vi "TestExec.Lookup Sequence XML Result Folder.vi"(9 "Seq Result Dirs":T1[](array[typedef]), 10 "Default Result Folder":path, 11 "Seq Name":string) -> (2 "None":bool, 3 "Result Folder":path)   [LabVIEW 2018]
uses:
  Common/Utils/TestExec/TestExec.WorkingDir.ctl
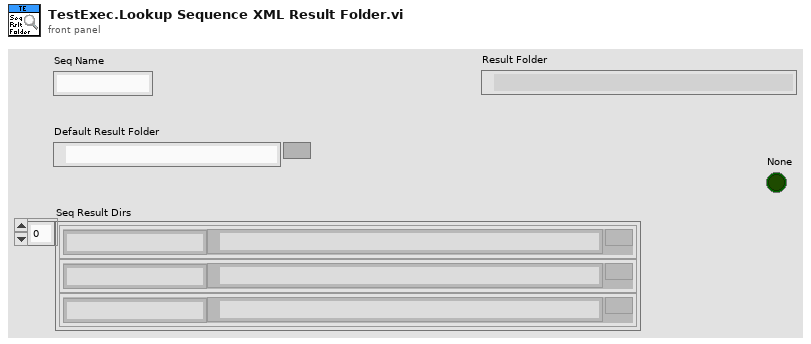
[diagram p1: front panel]
types:
  T1 = typedef "TestExec.WorkingDir.ctl" = cluster{"Name":string, "Path":path}
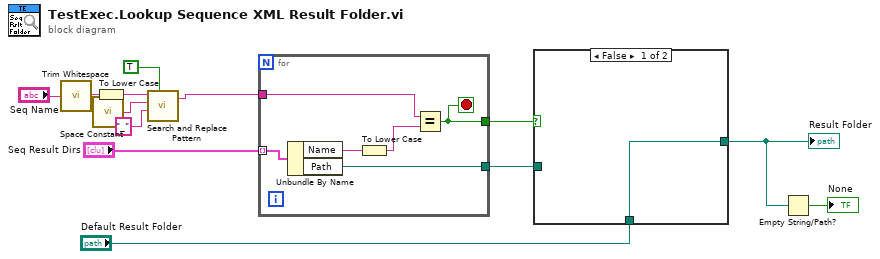
[diagram p0: block diagram]
diagram:
  n1 = call <vilib>:"Trim Whitespace.vi"("string"="Seq Name") -> ("trimmed string"=w2:string)  [unwired: 1 in]
  n2 = call <vilib>:"Space Constant.vi"() -> ("String"=w4:string)
  n3 = To Lower Case(string=w2) -> (all lower case string=w7:string)
  n4 = call <vilib>:"Search and Replace Pattern.vi"("string"=w7, "regular expression (\"\")"=w4, "replace string (\"\")"="_", "replace all? (F)"=TRUE) -> ("result string"=w6:string)  [unwired: 1 in, 1 out]
  n5 = for {
    tunnel: "Seq Result Dirs" -> [w19] mode=indexing
    tunnel: w6 -> [w17]
    tunnel: [w15] -> w12
    tunnel: [w14] -> w11
    stop <- w15 stop-if-true
    n6 = Unbundle By Name(w19) -> ("Name"=w18:string, "Path"=w14:path)
    n7 = To Lower Case(string=w18) -> (all lower case string=w16:string)
    n8 = Equal?(x=w17, y=w16) -> (x = y?=w15:bool)
  }
  n9 = case shown="False" w12 {
    tunnel: [w20 w21] -> w9
    tunnel: w11 -> [_ w21]
    tunnel: "Default Result Folder" -> [w20 _]
    frame False {
    }
    frame True {
    }
  }
  "Result Folder" <- w9
  n10 = Empty String/Path?(string/path=w9) -> (empty?=→"None":bool)
